vi "Close.vi"(7 "Monochromator in":T1, 8 "error in (no error)":errorcluster) -> (0 "error out":errorcluster)   [LabVIEW 2017, in "Monochromator.lvlib" / "Oriel (custom drivers).lvlib"]
uses:
  Oriel (custom drivers).lvlib
  Controls/Params.ctl
  C:/Users/Abigail/Documents/Imperial Optical software/Optical Software Code Simplified/Modules/Monochromator/Cornerstone.dll
  Cornerstone.dll
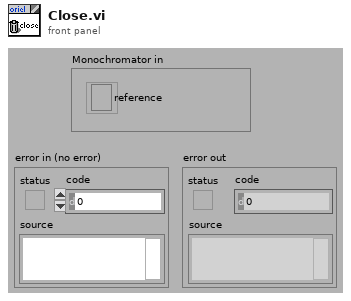
[diagram p1: front panel]
types:
  T1 = typedef "Monochromator.lvlib/Oriel (custom drivers).lvlib/Params.ctl" = cluster{"reference":refnum<k24>}
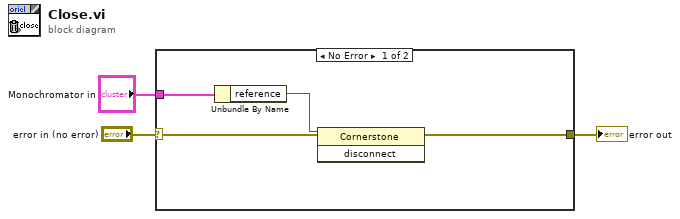
[diagram p0: block diagram]
diagram:
  n1 = case shown="No Error" "error in (no error)" {
    selector: "error in (no error)" -> [w7 w8]
    tunnel: [w6 w8] -> w2
    tunnel: "Monochromator in" -> [w4 _]
    frame No Error {
      n2 = Unbundle By Name(w4) -> ("reference"=w5:refnum<k24>)
      n3 = invoke class="Cornerstone" method="disconnect"(reference=w5, error in=w7) -> (error out=w6:errorcluster)  [unwired: 1 in, 2 out]
    }
    frame Error {
    }
  }
  "error out" <- w2
